vi "Get Key Value (String).vi"(5 "Key name":string, 6 "Default value":string, 7 "Section name":string, 8 "error in (no error)":errorcluster, 10 "Strip Whitespace? [T]":bool=TRUE, 11 "Carya Config in":refnum<class "Carya Config.lvclass">) -> (0 "error out":errorcluster, 1 "Found?":bool, 2 "Value":string, 3 "Carya Config out":refnum<class "Carya Config.lvclass">)   [LabVIEW 2013, in "Carya Config.lvclass"]
doc: "Copyright 2018, Carya Automatisering, Wiebe Walstra."
uses:
  Carya Config.lvclass
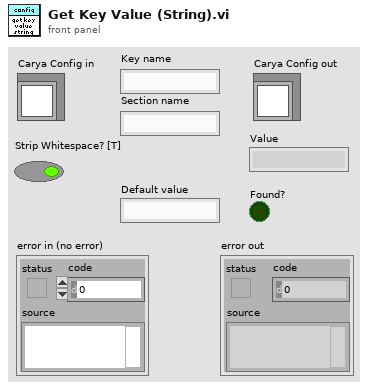
[diagram p1: front panel]
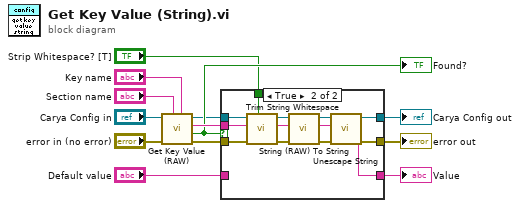
[diagram p0: block diagram]
diagram:
  n1 = call-dynamic "Get Key Value (RAW).vi"("Key name"="Key name", "Section name"="Section name", "error in (no error)"="error in (no error)", "Carya Config in"="Carya Config in") -> ("error out"=w12:errorcluster, "Found?"=w6:bool, "Value"=w7:string, "Carya Config out"=w3:refnum<class "Carya Config.lvclass">)  [unwired: 4 in]
  "Found?" <- w6
  n2 = case shown="True" w6 {
    tunnel: w12 -> [w15 w27]
    tunnel: [w15 w29] -> w8
    tunnel: w7 -> [_ w23]
    tunnel: "Default value" -> [w16 _]
    tunnel: [w16 w28] -> w5
    tunnel: w3 -> [w14 w24]
    tunnel: [w14 w26] -> w2
    tunnel: "Strip Whitespace? [T]" -> [_ w22]
    frame False {
    }
    frame True {
      n3 = call-dynamic "Trim String Whitespace.vi"("Strip Whitespace? [T]"=w22, "error in (no error)"=w27, "String"=w23, "Registry Object"=w24) -> ("error out"=w25:errorcluster, "Trimmed string"=w18:string, "Registry Object"=w20:refnum<class "Carya Config.lvclass">)  [unwired: 5 in]
      n4 = call-dynamic "String (RAW) To String.vi"("error in (no error)"=w25, "String (RAW)"=w18, "Registry Object"=w20) -> ("error out"=w21:errorcluster, "String"=w17:string, "Registry Object"=w19:refnum<class "Carya Config.lvclass">)  [unwired: 6 in]
      n5 = call-dynamic "Unescape String.vi"("error in (no error)"=w21, "String"=w17, "Registry Object"=w19) -> ("error out"=w29:errorcluster, "Unescaped string"=w28:string, "Registry Object"=w26:refnum<class "Carya Config.lvclass">)  [unwired: 6 in]
    }
  }
  "error out" <- w8
  "Carya Config out" <- w2
  "Value" <- w5
